vi "120_cm_Defense.vi"() -> (0 "String":string, 3 "Cluster":cluster{"State":T1, "Drive Control":T2} {"Drive Control"."Power (100)" min=-100 max=100})   [LabVIEW 2012, in "Serenity_mk2.lvrbt"]
uses:
  Serenity_mk2.lvrbt
  State_Typ.ctl
  auto_drive_TYP.ctl
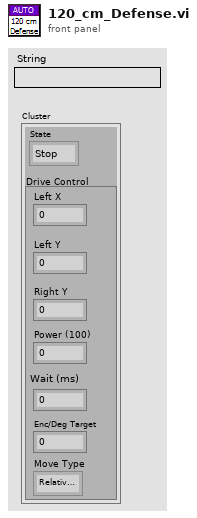
[diagram p1: front panel]
types:
  T1 = typedef "State_Typ.ctl" = enum16{"Stop", "Check for Position 3", "Check for Position 2", "Move", "Reset Enc", "Read Enc", "Lift", "Dump Close"}
  T2 = typedef "auto_drive_TYP.ctl" = cluster{"Left X":i8, "Left Y":i8, "Right Y":i8, "Power (100)":i8, "Wait (ms)":u32, "Enc/Deg Target":i32, "Move Type":enum16{"Relative Degrees", "Wait", "Encoder"}}
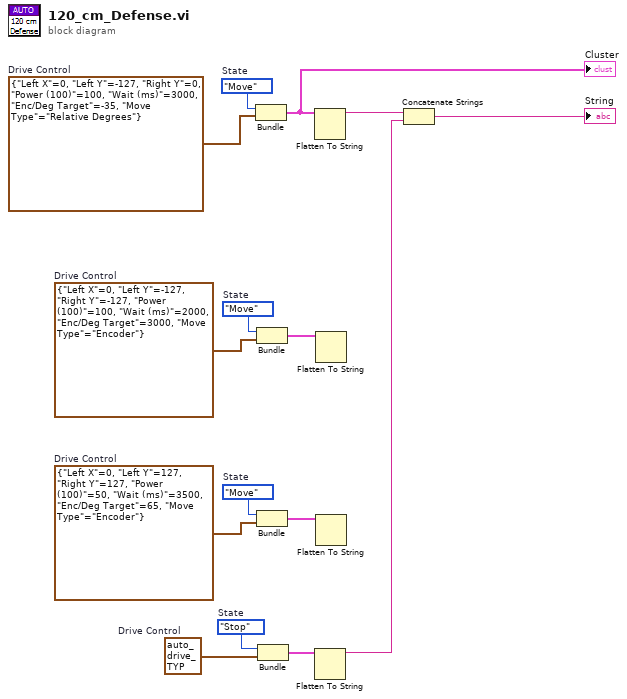
[diagram p0: block diagram]
diagram:
  w12 = T2 {"Left X"=0, "Left Y"=127, "Right Y"=127, "Power (100)"=50, "Wait (ms)"=3500, "Enc/Deg Target"=65, "Move Type"=enum."Encoder"}  # Drive Control
  w13 = State_Typ."Move"  # State
  w9 = T2 {"Left X"=0, "Left Y"=-127, "Right Y"=-127, "Power (100)"=100, "Wait (ms)"=2000, "Enc/Deg Target"=3000, "Move Type"=enum."Encoder"}  # Drive Control
  w10 = State_Typ."Move"  # State
  w5 = T2 {"Left X"=0, "Left Y"=0, "Right Y"=-127, "Power (100)"=40, "Wait (ms)"=700, "Enc/Deg Target"=-6500, "Move Type"=enum."Wait"}  # Drive Control
  w6 = State_Typ."Stop"  # State
  w1 = T2 {"Left X"=0, "Left Y"=-127, "Right Y"=0, "Power (100)"=100, "Wait (ms)"=3000, "Enc/Deg Target"=-35, "Move Type"=enum."Relative Degrees"}  # Drive Control
  w2 = State_Typ."Move"  # State
  n1 = Bundle("State"=w2, "Drive Control"=w1) -> (w3:cluster{"State":T1, "Drive Control":T2})  [unwired: 1 in]
  "Cluster" <- w3
  n2 = Bundle("State"=w10, "Drive Control"=w9) -> (w11:cluster{"State":T1, "Drive Control":T2})  [unwired: 1 in]
  n3 = Bundle("State"=w13, "Drive Control"=w12) -> (w14:cluster{"State":T1, "Drive Control":T2})  [unwired: 1 in]
  n4 = Bundle("State"=w6, "Drive Control"=w5) -> (w7:cluster{"State":T1, "Drive Control":T2})  [unwired: 1 in]
  n5 = Flatten To String(anything=w3) -> (data string=w4:string)  [unwired: 3 in, 2 out]
  n6 = Flatten To String(anything=w7) -> (data string=w15:string)  [unwired: 3 in, 2 out]
  n7 = Flatten To String(anything=w11) -> ()  [unwired: 3 in, 3 out]
  n8 = Flatten To String(anything=w14) -> ()  [unwired: 3 in, 3 out]
  n9 = Concatenate Strings(w4, w15) -> (→"String":string)
